vi "Bundle.vi"(8 "error in (no error)":errorcluster, 10 "Instrument DVR":refnum<data-value>, 11 "Instrument Owner in":refnum<class "Instrument Owner.lvclass">) -> (0 "error out":errorcluster, 3 "Instrument Owner out":refnum<class "Instrument Owner.lvclass">)   [LabVIEW 2020, in "Instrument Handler.lvlib" / "Instrument Owner.lvclass"]
doc: "Write the Instrument DVR to the Instrument Owner."
uses:
  Instrument Owner.lvclass
  Controls/Ctl_InstrumentSynchronicationCluster.ctl
  PPL/HDH.Actor Framework.Core.Instrument Driver.lvlibp/Instrument Driver/Controls/Ctl_ConnectionType.ctl
  PPL/HDH.Data.Generic.lvlibp/Synchronization/Notifier/Notifier.lvclass
  PPL/HDH.Actor Framework.Core.Actor.lvlibp/1abvi3w/vi.lib/ActorFramework/Message Enqueuer/Message Enqueuer.lvclass
  PPL/HDH.Actor Framework.Core.Sequencer.lvlibp/Sequencer Core/Sequencer Core.lvclass
  Instrument Owner.lvclass/Instrument Owner.ctl
  PPL/HDH.Actor Framework.Core.Instrument Driver.lvlibp/Instrument Driver/Instrument Driver.lvclass
  Instrument Handler.lvlib
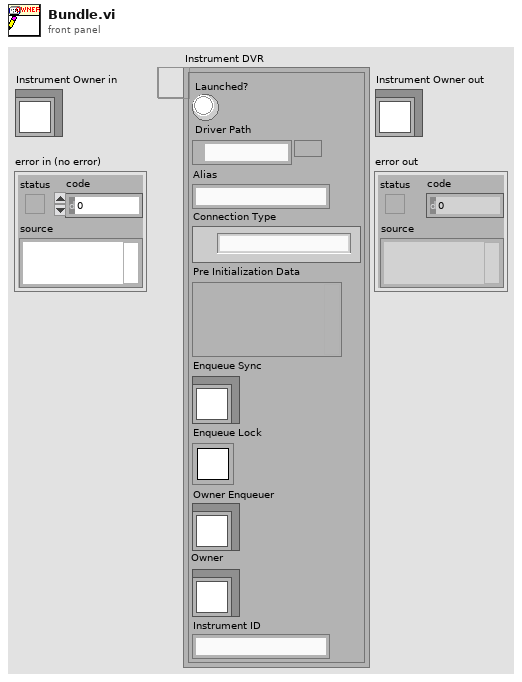
[diagram p1: front panel]
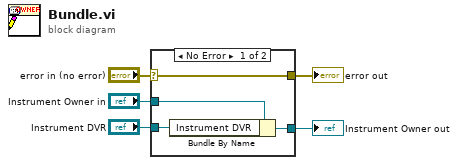
[diagram p0: block diagram]
diagram:
  n1 = case shown="No Error" "error in (no error)" {
    selector: "error in (no error)" -> [w9 w10]
    tunnel: [w9 w10] -> w4
    tunnel: [w7 w11] -> w2
    tunnel: "Instrument Owner in" -> [w8 w11]
    tunnel: "Instrument DVR" -> [w6 _]
    frame No Error {
      n2 = Bundle By Name(cluster=w8, "Instrument DVR"=w6) -> (w7:refnum<class "Instrument Owner.lvclass">)
    }
    frame Error {
    }
  }
  "error out" <- w4
  "Instrument Owner out" <- w2
